vi "Is Actor Public Method.vi"(8 "error in (no error)":errorcluster, 9 "Validation":T1, 11 "ProjectItem in":refnum<vi>) -> (0 "error out":errorcluster, 2 "Is Actor Public Method":bool, 3 "ProjectItem out":refnum<vi>, 4 "is actor interface?":bool)   [LabVIEW 2020, in "Message Maker Provider.lvlib"]
uses:
  Message Maker Provider.lvlib
  _Message Maker/Message Maker.lvlib
  AFPP Shared/Validation Mode.ctl
  AFPP Shared/AFPP Shared.lvlib
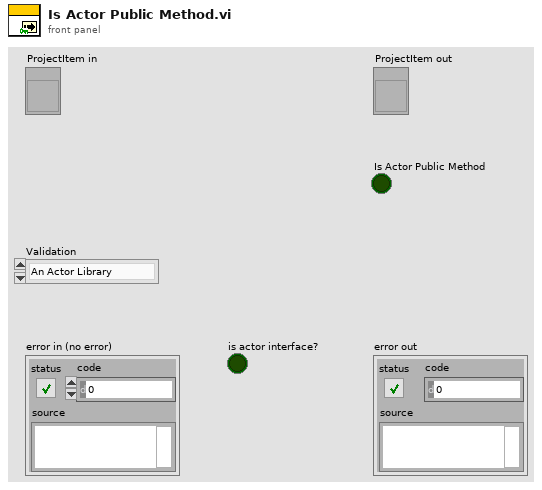
[diagram p1: front panel]
types:
  T1 = typedef "AFPP Shared.lvlib/Validation Mode.ctl" = enum16{"An Actor Library", "A Target Tag"}
  T2 = enum32{"invalid VI type", "Standard VI", "Control VI", "Global VI", "Polymorphic VI", "Configuration VI", "SubSystem", "Facade VI", "Method VI", "Statechart Diagram VI"}
  T3 = enum32{"invalid scope", "public", "private", "protected", "community"}
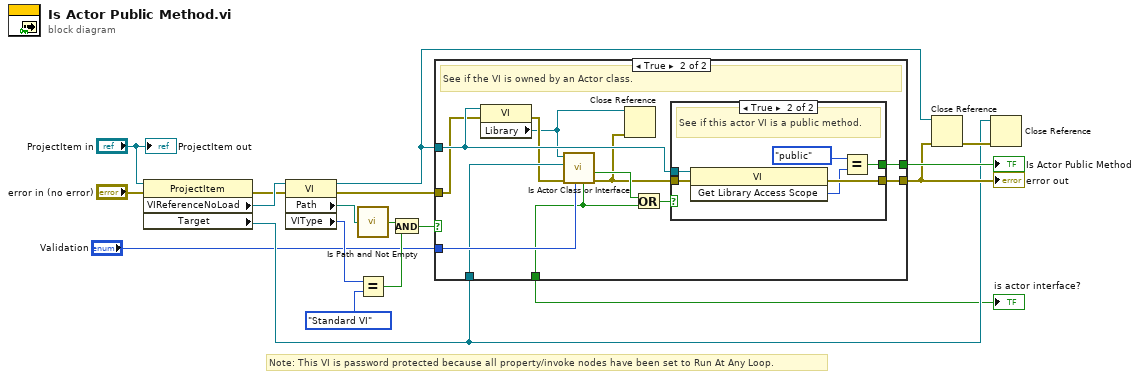
[diagram p0: block diagram]
diagram:
  # "Note: This VI is password protected because all property/invoke nodes have been set to Run At Any Loop."
  n1 = property class="ProjectItem"(reference="ProjectItem in", error in="error in (no error)") -> (error out=w16:errorcluster, "VIReferenceNoLoad"=w17:refnum<vi>, "Target"=w3:refnum<vi>)  [unwired: 1 out]
  n2 = property class="VI"(reference=w17, error in=w16) -> (reference out=w5:refnum<vi>, error out=w14:errorcluster, "Path"=w13:path, "VIType"=w12:T2)
  n3 = call <vilib>:"Is Path and Not Empty.vi"("path"=w13) -> ("Is Path and Not Empty?"=w10:bool)  [unwired: 4 in]
  n4 = Equal?(x=w12, y=T2."Standard VI") -> (x = y?=w9:bool)
  n5 = And(x=w10, y=w9) -> (x .and. y?=w8:bool)
  n6 = case shown="True" w8 {
    tunnel: [w19 w31] -> w6
    tunnel: w5 -> [_ w24]
    tunnel: [_ w30] -> w15
    tunnel: w14 -> [w19 w23]
    tunnel: w3 -> [_ w28]
    tunnel: "Validation" -> [_ w29]
    tunnel: [_ w25] -> w1
    frame False {
      # "Non standard VI, or VI not saved to disk."
    }
    frame True {
      # "See if the VI is owned by an Actor class."
      n7 = property class="VI"(reference=w24, error in=w23) -> (error out=w22:errorcluster, "Library"=w20:refnum<vi>)  [unwired: 1 out]
      n8 = call "Is Actor Class or Interface.vi"("Validation"=w29, "error in (no error)"=w22, "Target in"=w28, "LVClass Library in"=w20) -> ("error out"=w21:errorcluster, "is actor?"=w27:bool, "is actor interface?"=w25:bool)  [unwired: 4 in, 1 out]
      n9 = Close Reference(reference=w20, error in (no error)=w21) -> ()  [unwired: 1 out]
      n10 = Or(x=w27, y=w25) -> (x .or. y?=w26:bool)
      n11 = case shown="True" w26 {
        tunnel: [w32 w36] -> w31
        tunnel: [_ w34] -> w30
        tunnel: w24 -> [_ w38]
        tunnel: w21 -> [w32 w37]
        frame False {
          # "VI is not owned by an Actor class."
        }
        frame True {
          # "See if this actor VI is a public method."
          n12 = invoke class="VI" method="Get Library Access Scope"(reference=w38, error in=w37) -> (error out=w36:errorcluster, "Get Library Access Scope"=w35:T3)  [unwired: 1 in, 1 out]
          n13 = Equal?(x=T3."public", y=w35) -> (x = y?=w34:bool)
        }
      }
    }
  }
  "error out" <- w6
  "Is Actor Public Method" <- w15
  "is actor interface?" <- w1
  n14 = Close Reference(reference=w5, error in (no error)=w6) -> (error out=w4:errorcluster)
  n15 = Close Reference(reference=w3, error in (no error)=w4) -> ()  [unwired: 1 out]
  "ProjectItem out" <- "ProjectItem in"
